vi "AddDefect.vi"(7 "OpenTime (Now)":timestamp, 8 "error in":errorcluster, 10 "DefectId (GUID)":string, 11 "Datawarehouse in":refnum<class "Datawarehouse.lvclass">) -> (0 "error out":errorcluster, 2 "Defect":refnum<class "Defect.lvclass">, 3 "Datawarehouse out":refnum<class "Datawarehouse.lvclass">)   [LabVIEW 2021, in "ProligentXMLGenerator.lvlib" / "Datawarehouse.lvclass"]
doc: "Add a defect.\n\nA defect represents a physical problem with a UUT. When a defect exist on a UUT, the UUT is considered defective and needs to be repaired. A defect may be caused by a defective component, or by other causes (ex: component missing, solder missing, etc)."
uses:
  Datawarehouse.lvclass
  Datawarehouse.lvclass/Datawarehouse.ctl
  Failure/Defect/Defect.lvclass
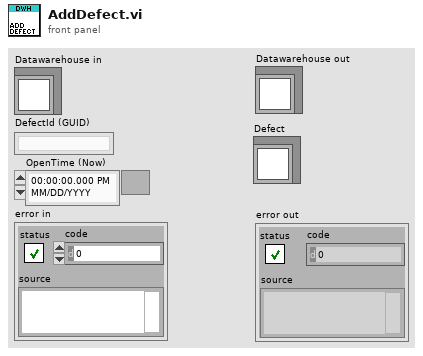
[diagram p1: front panel]
types:
  T1 = typedef "ProligentXMLGenerator.lvlib/Datawarehouse.lvclass/Data.ctl" = cluster{"DestinationFolder":path, "BaseFileName":string, "Document":refnum<k20>, "Defects":refnum<class "Defect.lvclass">[], "TopProcessRuns":refnum<class "ProcessRun.lvclass">[], "ProductUnits":refnum<class "ProductUnit.lvclass">[], "GenerationTime":refnum<class "DateTime.lvclass">, "DataSourceFingerprint":refnum<class "NonEmptyString_448.lvclass">, "IntegrationMetaData":refnum<class "NonEmptyString_2000.lvclass">, "TimeZoneInfoId":string}
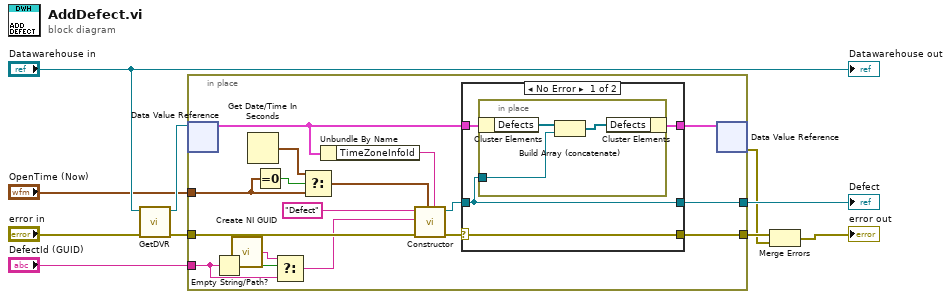
[diagram p0: block diagram]
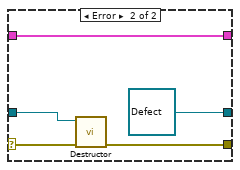
[diagram p2: hidden frame]
diagram:
  n1 = call "GetDVR.vi"("error in"="error in", "Datawarehouse"="Datawarehouse in") -> ("error out"=w5:errorcluster, "DVRReference"=w4:refnum<data-value>)  [unwired: 8 in]
  n2 = in-place "In Place Element Structure" {
    in-place-border: [w27] -> w6
    in-place-border: [w24] -> w10
    in-place-border: w5 -> [w23]
    in-place-border: "OpenTime (Now)" -> [w14]
    in-place-border: "DefectId (GUID)" -> [w18]
    n3 = in-place-dvr #1(w4) -> (w12:T1)  [unwired: 1 out]
    n4 = Empty String/Path?(string/path=w18) -> (empty?=w20:bool)
    n5 = call <vilib>:"Create NI GUID.vi"() -> ("NI GUID"=w19:string)
    n6 = Get Date/Time In Seconds() -> (seconds since 1Jan1904=w15:timestamp)
    n7 = Equal To 0?(x=w14) -> (x = 0?=w16:bool)
    n8 = Select(t=w19, s=w20, f=w18) -> (s? t:f=w17:string)
    n9 = Select(t=w15, s=w16, f=w14) -> (s? t:f=w13:timestamp)
    n10 = Unbundle By Name(w12) -> ("TimeZoneInfoId"=w11:string)
    n11 = call "Constructor.vi"("TimeZoneInfoId"=w11, "OpenTime"=w13, "error in"=w23, "DefectId"=w17, "Name"="Defect") -> ("error out"=w26:errorcluster, "Defect"=w25:refnum<class "Defect.lvclass">)  [unwired: 5 in]
    n12 = case shown="No Error" w26 {
      selector: w26 -> [w31 w38]
      tunnel: w12 -> [w30 w39]
      tunnel: w25 -> [w28 w36]
      tunnel: [w29 w39] -> w22
      tunnel: [w31 w37] -> w27
      tunnel: [w28 refnum<class "Defect.lvclass"> refnum ("Defect in")] -> w24
      frame No Error {
        n13 = in-place "In Place Element Structure" {
          in-place-border: w28 -> [w32]
          n14 = in-place-cluster #2(w30) -> ("Defects"=w34:refnum<class "Defect.lvclass">[])
          n15 = Build Array (concatenate)(w34, w32) -> (w33:refnum<class "Defect.lvclass">[])
          n16 = in-place-cluster #2("Defects"=w33) -> (w29:T1)
        }
      }
      frame Error {
        n17 = call "Destructor.vi"("error in"=w38, "Defect"=w36) -> ("error out"=w37:errorcluster)  [unwired: 9 in]
      }
    }
    n18 = in-place-dvr #1(w22) -> (w3:errorcluster)  [unwired: 1 out]
  }
  "Defect" <- w10
  n19 = Merge Errors(w6, w3) -> (→"error out":errorcluster)
  "Datawarehouse out" <- "Datawarehouse in"
